vi "Get IP Reg Types.vi"(10 "Version":T1, 11 "APU in":refnum<class "APU.lvclass">) -> (2 "IP Regs":variant[](array[variant]), 3 "APU out":refnum<class "APU.lvclass">)   [LabVIEW 2013, in "APU.lvclass"]
uses:
  APU.lvclass
  Bitfile Major Version.ctl
  Engine Simulation Session.lvclass
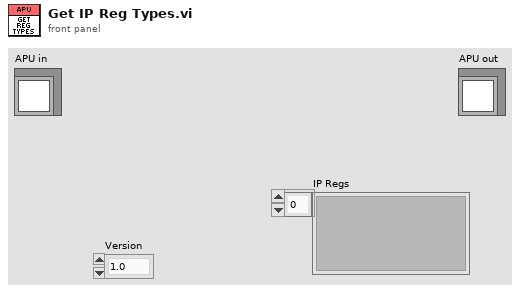
[diagram p1: front panel]
types:
  T1 = typedef "Engine Simulation Session.lvclass/Bitfile Major Version.ctl" = enum16{"1.0", "1.1", "1.2", "1.3"}
  T2 = cluster{"cycle start":fxp<+,2,2>, "crank start":u16, "stuck limit":fxp<+,18,18>}
  T3 = cluster{"start":fxp<+,17,17>, "stuck limit":fxp<+,18,18>}
  T4 = cluster{"crank":u16, "cycle":u16, "actual speed":fxp<+/-,23,2>}
  T5 = cluster{"desired speed":fxp<+/-,23,2>, "reset":bool}
  T6 = cluster{"acceleration":fxp<+,18,-20>, "max cycle":fxp<+,2,2>, "enable accel":bool}
  T7 = cluster{"acceleration":fxp<+,18,-20>, "enable accel":bool}
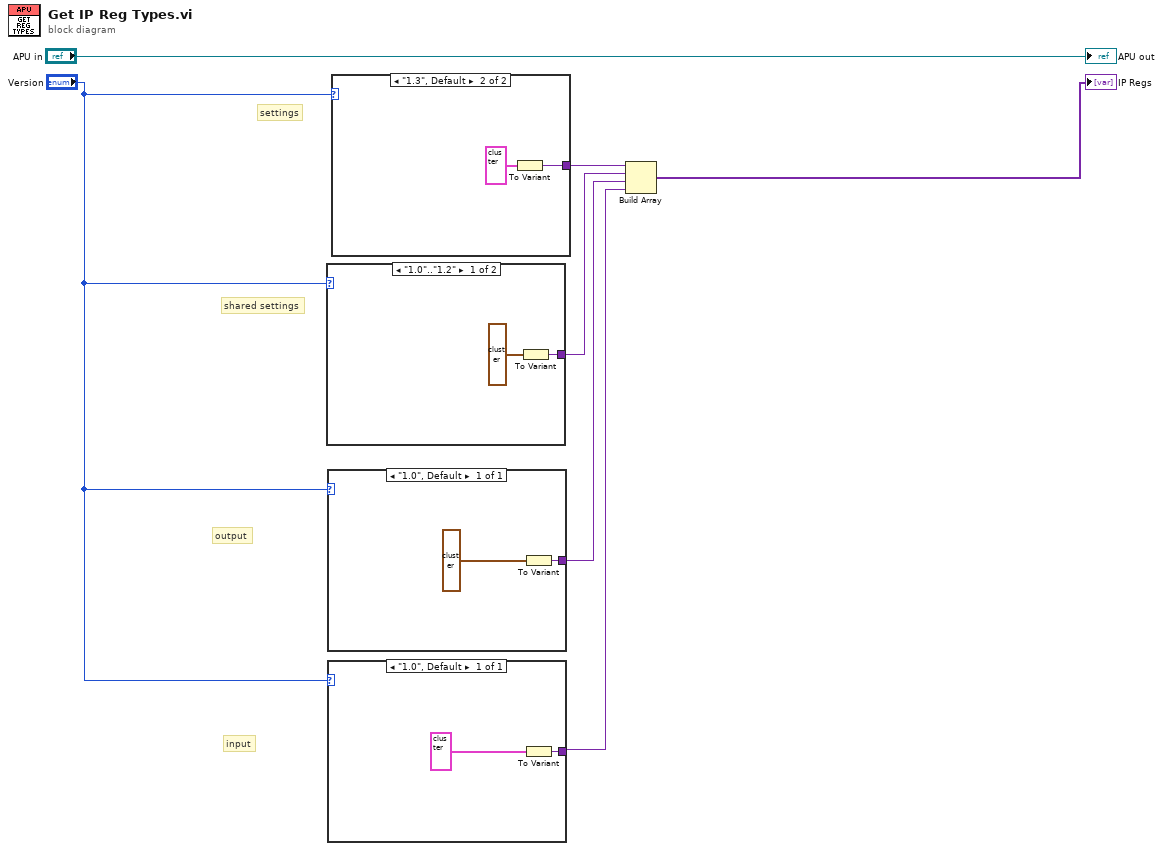
[diagram p0: block diagram]
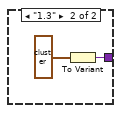
[diagram p2: hidden frame]
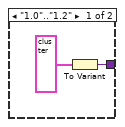
[diagram p3: hidden frame]
diagram:
  # "input"
  # "output"
  # "shared settings"
  # "settings"
  n1 = case shown="\"1.0\"..\"1.2\"" "Version" {
    tunnel: [w8 w11] -> w4
    frame "1.0".."1.2" {
      n2 = To Variant(anything=T2 {"cycle start"=0.0, "crank start"=0, "stuck limit"=0.0}) -> (Variant=w8:variant)
    }
    frame "1.3" {
      n3 = To Variant(anything=T3 {"start"=0.0, "stuck limit"=0.0} ("APU Shared Settings")) -> (Variant=w11:variant)
    }
  }
  n4 = case shown="\"1.0\", Default" "Version" {
    tunnel: [w13] -> w3
    frame "1.0", Default {
      n5 = To Variant(anything=T4 {"crank"=0, "cycle"=0, "actual speed"=0.0}) -> (Variant=w13:variant)
    }
  }
  n6 = case shown="\"1.0\", Default" "Version" {
    tunnel: [w15] -> w2
    frame "1.0", Default {
      n7 = To Variant(anything=T5 {"desired speed"=0.0, "reset"=FALSE}) -> (Variant=w15:variant)
    }
  }
  n8 = case shown="\"1.3\", Default" "Version" {
    tunnel: [w16 w18] -> w5
    frame "1.0".."1.2" {
      n9 = To Variant(anything=T6 {"acceleration"=0.0, "max cycle"=0.0, "enable accel"=FALSE}) -> (Variant=w16:variant)
    }
    frame "1.3", Default {
      n10 = To Variant(anything=T7 {"acceleration"=0.0, "enable accel"=FALSE} ("settings with acceleration")) -> (Variant=w18:variant)
    }
  }
  n11 = Build Array(w5, w4, w3, w2) -> (→"IP Regs":variant[])
  "APU out" <- "APU in"
